vi "SVFA Power Spectrum Subset (N Ch).vi"(0 "scaled signals [EU]":waveform(dbl)[](array[waveform]), 2 "window":T7=1 items=["None"=0, "Hanning"=1, "Hamming"=2, "Blackman-Harris"=3, "Exact Blackman"=4, "Blackman"=5, "Flat Top"=6, "4 Term B-Harris "=7, "7 Term B-Harris"=8, "Low Sidelobe"=9, "Force"=64, "Exponential"=65, "Blackman Nuttall"=11, "Triangle"=30, "Bartlett-Hanning"=31, "Bohman"=32, "Parzen"=33, "Welch"=34, "Kaiser"=60, "Dolph-Chebyshev"=61, "Gaussian"=62], 3 "frequency range":T9={"start frequency"=1000.0, "stop frequency"=2000.0} {"stop frequency" min=0.0 format="%.2f"; "start frequency" min=0.0 format="%.2f"}, 4 "dB On (T)":bool=TRUE, 5 "error in (no error)":errorcluster, 7 "averaging parameters":T8={"averaging mode"=enum."No averaging", "weighting mode"=enum."Exponential", "number of averages"=10, "linear mode"=enum."One shot"}, 9 "restart averaging (F)":bool) -> (11 "averaging done":bool, 13 "averages completed":dbl, 14 "power spectra [dB EU]":cluster{"f0":dbl, "df":dbl, "magnitude":dbl[]}[](array[cluster]) {"magnitude" format="%.2p"; "df" format="%.2p"; "f0" format="%.2p"}, 15 "unit labels":string[](array[string]), 18 "spectrum info":T1[](array[typedef]) {"x-axis units" items=["Time (s)"=0, "Frequency-CB (Hz)"=1, "Frequency-CPB (Hz)"=1248, "Frequency-Arbitrary (Hz)"=2357, "Quefrency (s)"=2, "Revolutions (rev)"=3, "Order"=4, "Speed (RPM)"=11, "Speed (rad/s)"=21, "Index"=65535]; "weighting filter" items=["Linear", "A-weighting", "B-weighting", "C-weighting", "ITU-R 468-4", "Dolby", "CCITT", "C-message", "Wb", "Wc", "Wd", "We", "Wf", "Wh", "Wj", "Wk", "Wm", "AES17 20 kHz lowpass", "AES17 40 kHz lowpass", "AES17 20 kHz highpass", "AES17 40 kHz highpass"]; "dB reference [EU]" format="%.2f"; "engineering units" items=["custom..."=0, "V"=1, "A"=21, "C"=30, "pC"=31, "s"=32, "-"=29, "Pa"=2, "N"=20, "g"=3, "m/s^2"=4, "m/s"=5, "m"=6, "mm/s"=12, "mm"=13, "micron/s"=14, "micron"=15, "in/s^2"=7, "in/s"=8, "in"=9, "mil/s"=10, "mil"=11, "rad/s^2"=16, "rad/s"=17, "rad"=18, "deg/s^2"=26, "deg/s"=27, "deg"=28, "RPM"=22, "cycle/s^2"=23, "Hz"=24, "cycle"=25, "strain"=19]; "spectral info"."window" items=["None "=0, "Hanning"=1, "Hamming"=2, "Blackman-Harris"=3, "Exact Blackman"=4, "Blackman"=5, "Flat Top"=6, "4 Term B-Harris "=7, "7 Term B-Harris"=8, "Low Sidelobe"=9, "Force - Exponential"=10, "Gaussian"=62]}, 19 "error out":errorcluster)   [LabVIEW 2017]
doc: "Computes a subset of the power spectrum of <B>scaled signal [EU]</B>. The subset is defined by <B>frequency range</B>. Each block of data corresponds to a single FFT block and has to be passed individually to this VI. Wire data to the <B>scaled signal [EU]</B> input to determine the polymorphic instance to use or manually select the instance."
uses:
  <vilib>/addons/_NISVFA/_Shared subVIs/Controls/svc_Window.ctl
  <vilib>/addons/_NISVFA/_Shared subVIs/Controls/svc_Spectrum Info.ctl
  <vilib>/addons/_NISVFA/_Shared subVIs/Controls/svc_X-Axis Units.ctl
  <vilib>/addons/_NISVFA/_Shared subVIs/Controls/svc_Spectrum Type.ctl
  <vilib>/addons/_NISVFA/_Shared subVIs/Controls/svc_Engineering Units Text Ring.ctl
  <vilib>/addons/_NISVFA/_Shared subVIs/Controls/svc_Weighting Filter Text Ring.ctl
  <vilib>/addons/_NISVFA/_Shared subVIs/Controls/svc_Complimentary Spectrum Units.ctl
  <vilib>/addons/_NISVFA/_Shared subVIs/Windowing/svfa_Scaled Time Domain Window (1 Ch).vi
  <vilib>/addons/_NISVFA/_Shared subVIs/Spectrum Info/svfa_Build Spectrum Info.vi
  <vilib>/addons/_NISVFA/_Shared subVIs/Spectrum Averaging/svfa_Reset Averaging State Info.vi
  <vilib>/addons/_NISVFA/_Shared subVIs/Spectrum Averaging/svfa_Average Array with Avg Checks (complex) No State.vi
  <vilib>/addons/_NISVFA/_Shared subVIs/Common/svc_Complex to Mag2 Array.vi
  <vilib>/addons/_NISVFA/_Shared subVIs/Spectrum Averaging/svfa_Average Array with Avg Checks (real) No State.vi
  <vilib>/addons/_NISVFA/_Shared subVIs/Windowing/svfa_Scaled Time Domain Window (Array).vi
  <vilib>/addons/_NISVFA/_Shared subVIs/Common/svc_Get SV Channel Info.vi
  <vilib>/addons/_NISVFA/_Shared subVIs/Common/svc_Spectrum Units.vi
  <vilib>/addons/_NISVFA/_Shared subVIs/Spectrum Averaging/svfa_Average Array (complex) No State.vi
  <vilib>/addons/_NISVFA/_Shared subVIs/Spectrum Averaging/svfa_Average Array (real) No State.vi
  <vilib>/Analysis/4window.llb/Force Window.vi
  <vilib>/Analysis/4window.llb/Force Window (DBL).vi
  <vilib>/Analysis/4window.llb/Exponential Window.vi
  <vilib>/Analysis/4window.llb/Exponential Window (DBL).vi
  <vilib>/addons/_NISVFA/_Shared subVIs/Spectrum Averaging/svfa_No Average Array (complex).vi
  <vilib>/addons/_NISVFA/_Shared subVIs/Spectrum Averaging/svfa_Average Array (complex).vi
  <vilib>/addons/_NISVFA/_Shared subVIs/Spectrum Averaging/svfa_No Average Array (real).vi
  <vilib>/addons/_NISVFA/_Shared subVIs/Spectrum Averaging/svfa_Average Array (real).vi
  <vilib>/addons/_NISVFA/_Shared subVIs/Spectrum Averaging/svfa_Peak Hold Array.vi
  <vilib>/addons/_NISVFA/_Shared subVIs/Common/svc_Get Weighting Enum and Labels.vi
  <vilib>/addons/_NISVFA/_Shared subVIs/Common/svc_Unit Label Lexical Class.vi
  <vilib>/addons/_NISVFA/_Shared subVIs/Common/svc_Engineering Units to Unit Label.vi
  <vilib>/addons/_NISVFA/_Shared subVIs/Common/svc_Format Value (DBL).vi
  <vilib>/addons/_NISVFA/_Shared subVIs/Common/svc_Channel Info to Spectrum Info.vi
  <vilib>/addons/_NISVFA/_Shared subVIs/Common/svc_Unit Label to Engineering Units.vi
  <vilib>/Utility/error.llb/Error Cluster From Error Code.vi
  <vilib>/Analysis/0measdsp.llb/Scaled Time Domain Window.vi
  <vilib>/Analysis/0measdsp.llb/Scaled Time Domain Window (DBL).vi
  <vilib>/addons/_NISVFA/_Spectrum Processing/subVIs/svfa_Spectrum Info Window to windowTd Type Def.vi
  <vilib>/addons/_NISVFA/_Shared subVIs/Common/svc_Window Parameters.vi
  <vilib>/addons/_NISVFA/_Shared subVIs/Common/svc_Get Window Info.vi
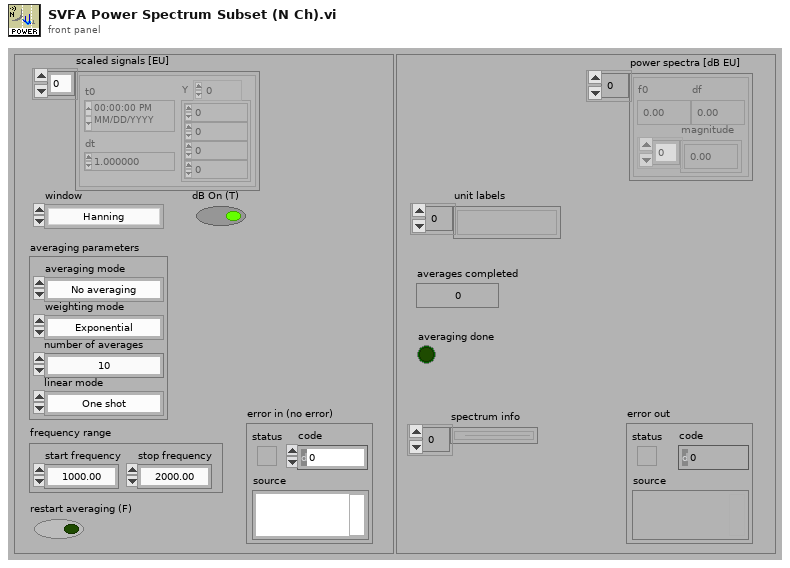
[diagram p1: front panel]
types:
  T1 = typedef "svc_Spectrum Info.ctl" = cluster{"channel name":string, "description":string, "x-axis units":T2, "spectral info":cluster{"spectrum type":T3, "linear/dB":enum16{"linear", "dB"}, "window":u16, "window size":i32, "FFT size":i32}, "engineering units":T4, "custom label":string, "dB reference [EU]":dbl, "peak units":enum16{"rms", "peak", "peak-peak"}, "weighting filter":T5, "spectral density?":bool, "unit label":string, "spectrum skewed?":bool, "complimentary spectrum units":T6}
  T2 = typedef "svc_X-Axis Units.ctl" = u16
  T3 = typedef "svc_Spectrum Type.ctl" = enum16{"FFT Spectrum [complex]", "Amplitude [Magnitude]", "Power [Magnitude^2]", "Cross Spectrum [complex]", "Frequency Response [Complex]"}
  T4 = typedef "svc_Engineering Units Text Ring.ctl" = u16
  T5 = typedef "svc_Weighting Filter Text Ring.ctl" = u16
  T6 = typedef "svc_Complimentary Spectrum Units.ctl" = enum16{"none", "radians", "degrees", "cycles", "imaginary"}
  T7 = typedef "svc_Window.ctl" = u32
  T8 = cluster{"averaging mode":enum16{"No averaging", "Vector averaging", "RMS averaging", "Peak hold"}, "weighting mode":enum16{"Linear", "Exponential"}, "number of averages":u32, "linear mode":enum16{"One shot", "Auto restart"}}
  T9 = cluster{"start frequency":dbl, "stop frequency":dbl}
  T10 = enum16{"Restart processing", "Continue processing", "Skip processing"}
  T11 = cluster{"complex FFT":cdb[], "real FFT":dbl[], "f0":dbl, "df":dbl, "averages completed":dbl, "averaging parameters":cluster{"averaging mode":enum16{"No averaging", "Vector averaging", "RMS averaging", "Peak hold"}, "weighting mode":enum16{"Linear", "Exponential"}, "number of averages":u32, "linear mode":enum16{"One shot", "Auto restart"}}}[]
  T12 = enum16{"No averaging", "Vector averaging", "RMS averaging", "Peak hold"}
  T13 = cluster{"complex FFT":cdb[], "real FFT":dbl[], "f0":dbl, "df":dbl, "averages completed":dbl, "averaging parameters":cluster{"averaging mode":enum16{"No averaging", "Vector averaging", "RMS averaging", "Peak hold"}, "weighting mode":enum16{"Linear", "Exponential"}, "number of averages":u32, "linear mode":enum16{"One shot", "Auto restart"}}}
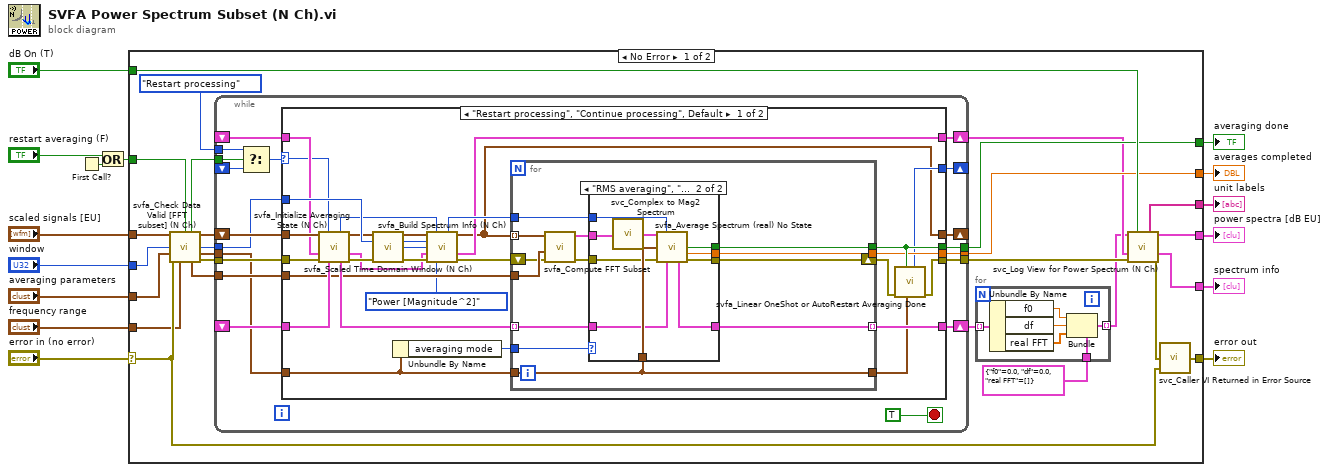
[diagram p0: block diagram]
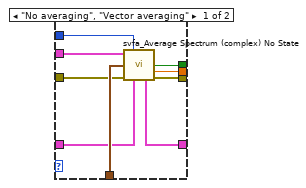
[diagram p2: hidden frame]
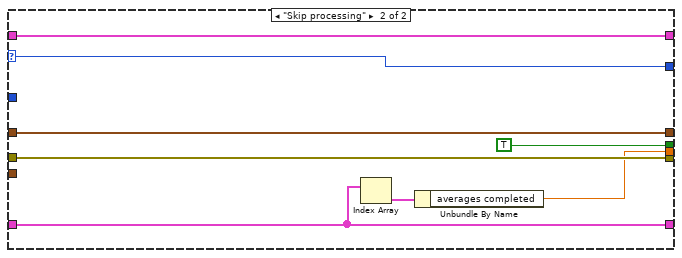
[diagram p3: hidden frame]
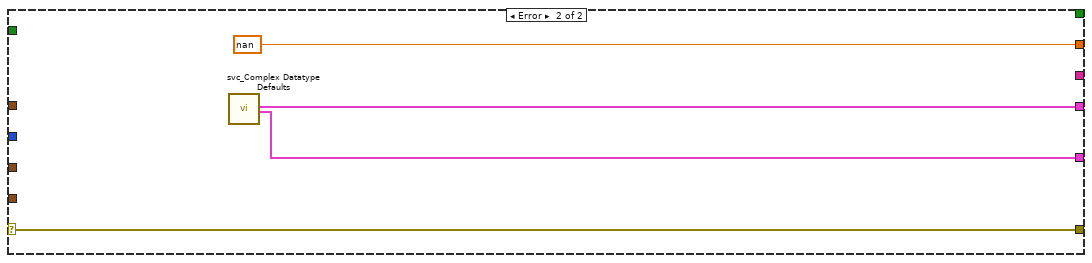
[diagram p4: hidden frame]
diagram:
  n1 = First Call?() -> (First Call?: T/F=w3:bool)
  n2 = Or(x="restart averaging (F)", y=w3) -> (x .or. y?=w2:bool)
  n3 = case shown="No Error" "error in (no error)" {
    selector: "error in (no error)" -> [w31 w140]
    tunnel: w2 -> [w39 _]
    tunnel: [w20 nan ("Averaged So-far")] -> w15
    tunnel: [w19 _] -> w14
    tunnel: [w36 w138] -> w9
    tunnel: [w33 w140] -> w13
    tunnel: "averaging parameters" -> [w38 _]
    tunnel: "frequency range" -> [w30 _]
    tunnel: "scaled signals [EU]" -> [w41 _]
    tunnel: "window" -> [w40 _]
    tunnel: [w35 _] -> w6
    tunnel: "dB On (T)" -> [w37 _]
    tunnel: [w32 w137] -> w4
    frame No Error {
      n4 = call <vilib>:"svfa_Check Data Valid [FFT subset] (N Ch).vi"("scaled signals"=w41, "restart averaging (F)"=w39, "window"=w40, "averaging parameters"=w38, "error in (no error)"=w31, "frequency range in"=w30) -> ("restart averaging"=w22:bool, "dup scaled signals"=w28:waveform(dbl)[], "window"=w25:u16, "dup averaging parameters"=w24:T8, "frequency range out"=w26:T9, "error out"=w27:errorcluster)  [unwired: 4 in]
      n5 = while {
        shift-left: _ -> [w56]
        shift-right: [w57] -> w29
        tunnel: [w63] -> w20
        tunnel: [w64] -> w19
        tunnel: [w65] -> w21
        tunnel: w27 -> [w61]
        tunnel: w26 -> [w66]
        shift-right: [w59] -> w18
        shift-left: _ -> [w58]
        shift-right: [w55] -> _
        shift-left: _ -> [w54]
        tunnel: w25 -> [w52]
        tunnel: w24 -> [w51]
        tunnel: T10."Restart processing" ("processing control in") -> [w50]
        tunnel: w22 -> [w49]
        shift-right: [w48] -> _
        shift-left: w28 -> [w62]
        stop <- TRUE stop-if-true
        n6 = Select(t=w50, s=w49, f=w54) -> (s? t:f=w53:T10)
        n7 = case shown="\"Restart processing\", \"Continue processing\", Default" w53 {
          selector: w53 -> [w70 w134]
          tunnel: w66 -> [w79 _]
          tunnel: w51 -> [w89 _]
          tunnel: [w69 w130] -> w59
          tunnel: [w95 w132] -> w57
          tunnel: [w88 w135] -> w65
          tunnel: [w93 TRUE ("averaging done?")] -> w64
          tunnel: [w92 w133] -> w63
          tunnel: w62 -> [w86 w129]
          tunnel: w61 -> [w85 w135]
          tunnel: w58 -> [w80 w130]
          tunnel: w56 -> [w84 w132]
          tunnel: [w90 w134] -> w55
          tunnel: w52 -> [w91 _]
          tunnel: [w67 w129] -> w48
          frame "Restart processing", "Continue processing", Default {
            n8 = call <vilib>:"svfa_Initialize Averaging State (N Ch).vi"("Windowed Waveform(s)"=w86, "processing control in"=w70, "spectra info in"=w80, "error in (no error)"=w85, "state info"=w84) -> ("processing control out"=w68:T10, "Windowed Waveform(s)"=w82:waveform(dbl)[], "spectra info out"=w71:T1[], "state info"=w83:T11, "error out"=w81:errorcluster)  [unwired: 6 in]
            n9 = call <vilib>:"svfa_Scaled Time Domain Window (N Ch).vi"("Scaled signal(s)"=w82, "window"=w91, "error in (no error)"=w81) -> ("Windowed Waveform(s)"=w78:waveform(dbl)[], "window"=w75:T7, "window length"=w74:i32, "error out"=w73:errorcluster)  [unwired: 8 in, 1 out]
            n10 = Unbundle By Name(w89) -> ("averaging mode"=w96:T12)
            n11 = call <vilib>:"svfa_Build Spectrum Info (N Ch).vi"("scaled signal(s)"=w78, "processing control in"=w68, "window"=w75, "window size"=w74, "spectra info in"=w71, "error in (no error)"=w73, "spectrum type"=svc_Spectrum_Type."Power [Magnitude^2]" ("spectrum type 2")) -> ("dup processing control"=w77:T10, "dup scaled signals"=w67:waveform(dbl)[], "spectra info out"=w69:T1[], "error out"=w72:errorcluster)  [unwired: 5 in]
            n12 = for {
              tunnel: w96 -> [w109]
              tunnel: [w102] -> w95 mode=indexing
              tunnel: [w107] -> w93
              tunnel: [w106] -> w92
              tunnel: w77 -> [w105]
              tunnel: w89 -> [w103]
              tunnel: w83 -> [w104] mode=indexing
              tunnel: [w103] -> w87
              shift-right: [w108] -> w94
              shift-left: w72 -> [w99]
              tunnel: w79 -> [w100]
              tunnel: w67 -> [w101] mode=indexing
              n13 = call <vilib>:"svfa_Compute FFT Subset.vi"("error in (no error)"=w99, "frequency range"=w100, "windowed signal"=w101) -> ("error out"=w98:errorcluster, "FFT spectrum [Vrms]"=w97:cluster{"f0":dbl, "df":dbl, "spectrum":cdb[]})  [unwired: 7 in]
              n14 = case shown="\"RMS averaging\", \"Peak hold\"" w109 {
                tunnel: w103 -> [w118 w124]
                tunnel: [w110 w121] -> w102
                tunnel: [w117 w127] -> w108
                tunnel: [w116 w128] -> w107
                tunnel: w98 -> [w111 w120]
                tunnel: w105 -> [w114 w123]
                tunnel: [w115 w126] -> w106
                tunnel: w104 -> [w113 w122]
                tunnel: w97 -> [w112 w119]
                frame "No averaging", "Vector averaging" {
                  n15 = call <vilib>:"svfa_Average Spectrum (complex) No State.vi"("spectrum"=w112, "processing control"=w114, "averaging parameters"=w118, "error in (no error)"=w111, "averaging state info in"=w113) -> ("averaging done"=w116:bool, "averages completed"=w115:dbl, "averaging state info out"=w110:T13, "error out"=w117:errorcluster)  [unwired: 5 in, 2 out]
                }
                frame "RMS averaging", "Peak hold" {
                  n16 = call <vilib>:"svc_Complex to Mag2 Spectrum.vi"("complex spectrum"=w119) -> ("power spectrum"=w125:cluster{"f0":dbl, "df":dbl, "spectrum":dbl[]})  [unwired: 4 in]
                  n17 = call <vilib>:"svfa_Average Spectrum (real) No State.vi"("spectrum"=w125, "processing control"=w123, "averaging parameters"=w124, "error in (no error)"=w120, "averaging state info in"=w122) -> ("averaging done"=w128:bool, "averages completed"=w126:dbl, "averaging state info out"=w121:T13, "error out"=w127:errorcluster)  [unwired: 5 in, 2 out]
                }
              }
            }
            n18 = call <vilib>:"svfa_Linear OneShot or AutoRestart Averaging Done.vi"("averaging parameters"=w87, "averaging done"=w93, "error in (no error)"=w94) -> ("error out"=w88:errorcluster, "processing control"=w90:T10)  [unwired: 7 in]
          }
          frame "Skip processing" {
            n19 = Index Array(array=w132) -> (element=w131:T13)  [unwired: 1 in]
            n20 = Unbundle By Name(w131) -> ("averages completed"=w133:dbl)
          }
        }
      }
      n21 = for {
        tunnel: w29 -> [w44] mode=indexing
        tunnel: [w43] -> w17 mode=indexing
        tunnel: cluster{"f0":dbl, "df":dbl, "real FFT":dbl[]} {"f0"=0.0, "df"=0.0, "real FFT"=[]} ("cluster") -> [w42]
        n22 = Unbundle By Name(w44) -> ("f0"=w45:dbl, "df"=w46:dbl, "real FFT"=w47:dbl[])
        n23 = Bundle(cluster=w42, "f0"=w45, "df"=w46, "real FFT"=w47) -> (w43:cluster{"f0":dbl, "df":dbl, "real FFT":dbl[]})
      }
      n24 = call <vilib>:"svc_Log View for Power Spectrum (N Ch).vi"("Power Spectra [EU^2 rms]"=w17, "dB On (F)"=w37, "spectra info in"=w18, "error in (no error)"=w21) -> ("unit label(s)"=w35:string[], "Power Spectra [EU^2 rms]"=w36:cluster{"f0":dbl, "df":dbl, "spectrum":dbl[]}[], "spectra info out"=w32:T1[], "error out"=w34:errorcluster)  [unwired: 8 in]
      n25 = call <vilib>:"svc_Caller VI Returned in Error Source.vi"("warning input to caller"=w31, "error in (no error)"=w34) -> ("error out"=w33:errorcluster)  [unwired: 3 in]
    }
    frame Error {
      n26 = call <vilib>:"svc_Complex Datatype Defaults.vi"() -> ("empty array of spectra"=w138:cluster{"f0":dbl, "df":dbl, "magnitude":dbl[]}[], "empty array of spectrum info"=w137:T1[])  [unwired: 11 in, 7 out]
    }
  }
  "averages completed" <- w15
  "averaging done" <- w14
  "error out" <- w13
  "power spectra [dB EU]" <- w9
  "unit labels" <- w6
  "spectrum info" <- w4
